vi "TypeDescriptor_SetName.vi"(10 "name":string, 11 "type descriptor":i16[](array[numeric]) format="%04x") -> (1 "named?":bool, 2 "name out":string, 3 "type descriptor dup":i16[](array[numeric]) format="%04x")   [LabVIEW 2013, in "OpenDescriptor.lvlib"]
uses:
  OpenDescriptor.lvlib
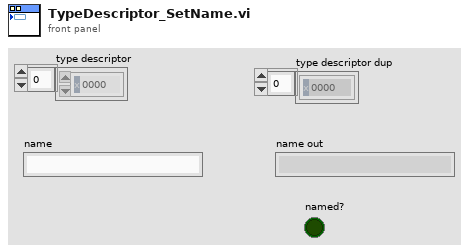
[diagram p1: front panel]
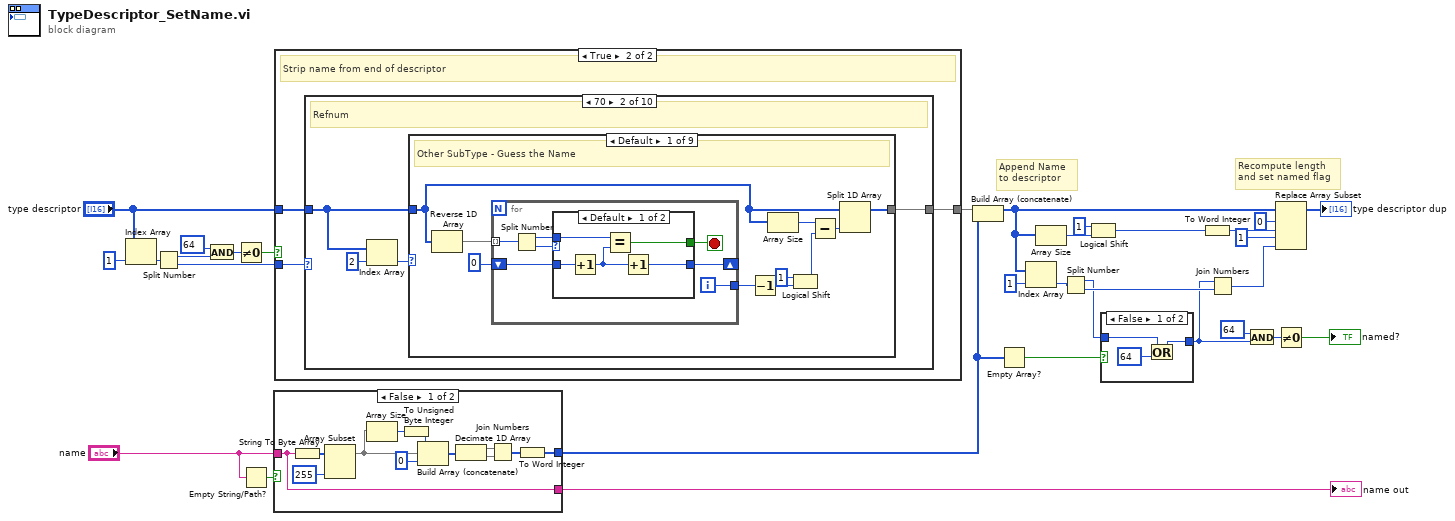
[diagram p0: block diagram]
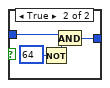
[diagram p2: hidden frame]
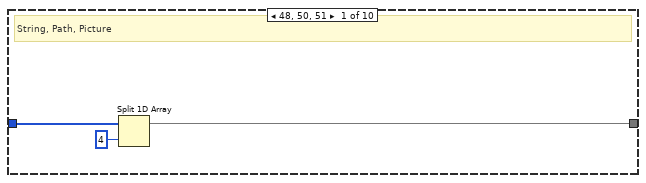
[diagram p5: hidden frame]
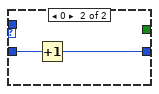
[diagram p6: hidden frame]
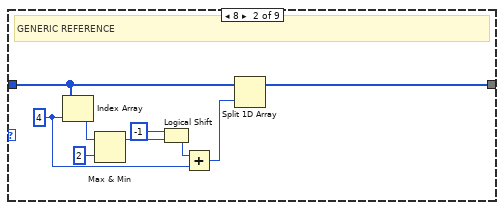
[diagram p7: hidden frame]
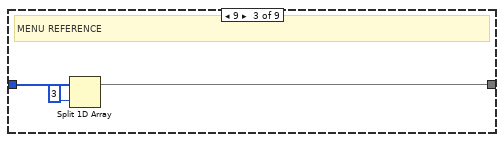
[diagram p8: hidden frame]
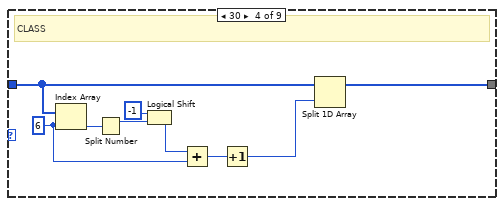
[diagram p9: hidden frame]
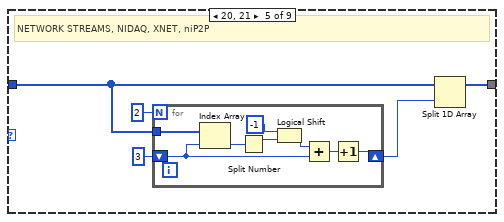
[diagram p10: hidden frame]
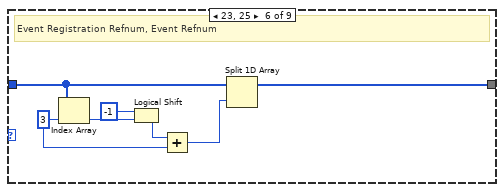
[diagram p11: hidden frame]
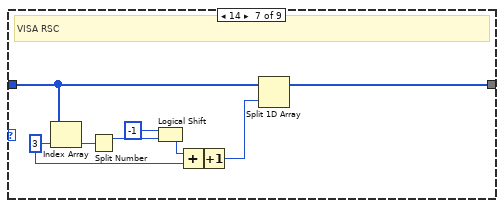
[diagram p12: hidden frame]
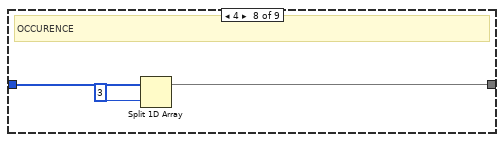
[diagram p13: hidden frame]
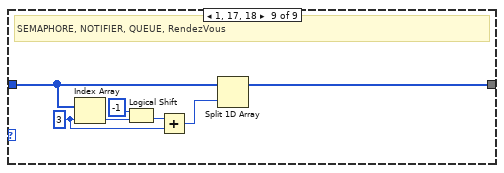
[diagram p14: hidden frame]
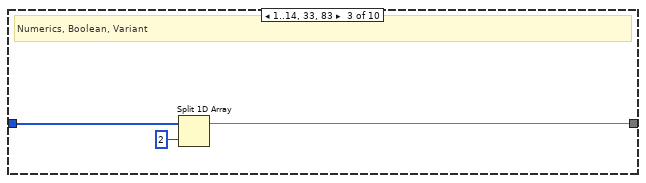
[diagram p15: hidden frame]
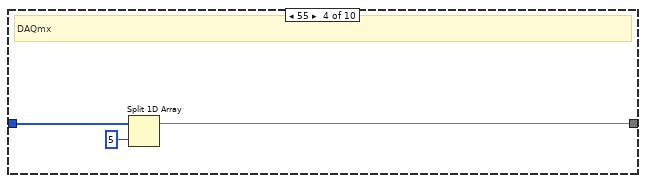
[diagram p16: hidden frame]
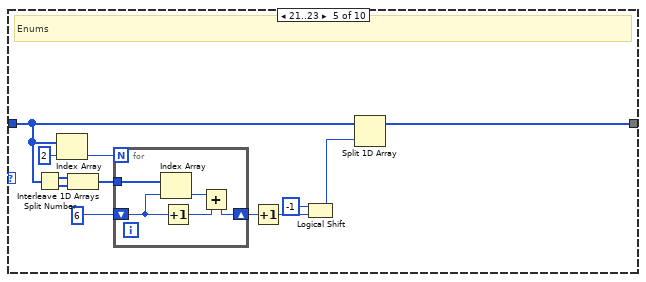
[diagram p17: hidden frame]
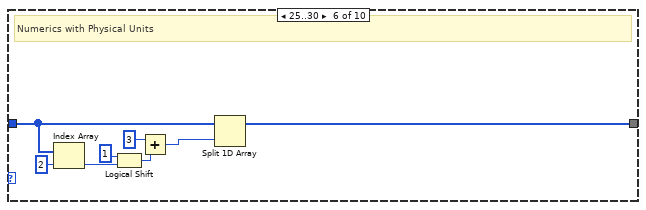
[diagram p18: hidden frame]
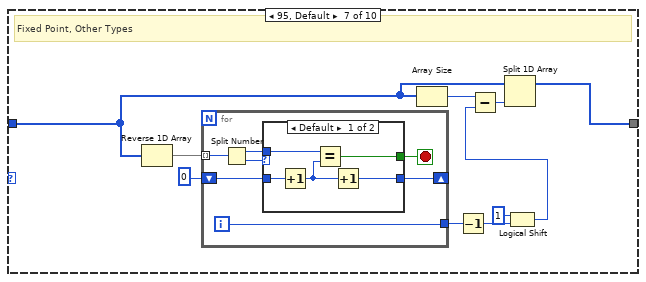
[diagram p19: hidden frame]
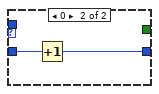
[diagram p20: hidden frame]
diagram:
  # "Recompute length\nand set named flag"
  # "Append Name\nto descriptor"
  n1 = Index Array(array="type descriptor", index=1) -> (element=w31:i16)
  n2 = Split Number(x=w31) -> (hi(x)=w26:u8, lo(x)=w28:u8)
  n3 = And(x=u8 64, y=w26) -> (x .and. y?=w24:u8)
  n4 = Not Equal To 0?(x=w24) -> (x != 0?=w29:bool)
  n5 = Empty String/Path?(string/path="name") -> (empty?=w22:bool)
  n6 = case shown="False" w22 {
    tunnel: [w33 _] -> w8
    tunnel: "name" -> [w32 _]
    tunnel: [w32 _] -> w1
    frame False {
      n7 = String To Byte Array(string=w32) -> (unsigned byte array=w38:u8[])
      n8 = Array Subset(array=w38, length=255) -> (w37:u8[])  [unwired: 1 in]
      n9 = Array Size(array=w37) -> (size(s)=w36:i32)
      n10 = To Unsigned Byte Integer(number=w36) -> (unsigned 8bit integer=w35:u8)
      n11 = Build Array (concatenate)(w35, w37, u8 0) -> (w42:u8[])
      n12 = Decimate 1D Array(w42) -> (w41:u8[], w40:u8[])
      n13 = Join Numbers(hi=w41, lo=w40) -> ((hi.lo)=w34:u16[])
      n14 = To Word Integer(number=w34) -> (16bit integer=w33:i16[])
    }
    frame True {
    }
  }
  "name out" <- w1
  n15 = case shown="True" w29 {
    tunnel: w28 -> [_ w46]
    tunnel: [w44 w45] -> w9
    tunnel: "type descriptor" -> [w44 w47]
    frame False {
    }
    frame True {
      # "Strip name from end of descriptor"
      n16 = case shown="70" w46 {
        tunnel: w47 -> [w50 w52 w140 w143 w147 w164 w174 w195 w207 w215]
        tunnel: [w48 w51 w139 w142 w145 w162 w175 w194 w208 w214] -> w45
        frame 48, 50, 51 {
          # "String, Path, Picture"
          n17 = Split 1D Array(array=w50, index=4) -> (first subarray=w48:i16[])  [unwired: 1 out]
        }
        frame 112 {
          # "Refnum"
          n18 = Index Array(array=w52, index=2) -> (element=w53:i16)
          n19 = case shown="Default" w53 {
            tunnel: w52 -> [w60 w81 w90 w92 w102 w115 w121 w131 w133]
            tunnel: [w59 w79 w88 w91 w101 w113 w122 w129 w132] -> w51
            frame Default {
              # "Other SubType - Guess the Name"
              n20 = Reverse 1D Array(array=w60) -> (reversed array=w63:i16[])
              n21 = for {
                tunnel: w63 -> [w66] mode=indexing
                shift-right: [w68] -> _
                shift-left: u8 0 ("hi(x)") -> [w69]
                tunnel: [w65] -> w55
                i -> [w65]
                stop <- w67 stop-if-true
                n22 = Split Number(x=w66) -> (hi(x)=w70:u8, lo(x)=w71:u8)
                n23 = case shown="Default" w71 {
                  tunnel: [w72 _] -> w67
                  tunnel: w70 -> [w76 _]
                  tunnel: w69 -> [w75 w78]
                  tunnel: [w73 w77] -> w68
                  frame Default {
                    n24 = Increment(x=w75) -> (x+1=w74:u8)
                    n25 = Equal?(x=w76, y=w74) -> (x = y?=w72:bool)
                    n26 = Increment(x=w74) -> (x+1=w73:u8)
                  }
                  frame 0 {
                    n27 = Increment(x=w78) -> (x+1=w77:u8)
                  }
                }
              }
              n28 = Decrement(x=w55) -> (x-1=w57:i32)
              n29 = Array Size(array=w60) -> (size(s)=w62:i32)
              n30 = Logical Shift(y=i16 1, x=w57) -> (x << y=w56:i32)
              n31 = Subtract(x=w62, y=w56) -> (x-y=w61:i32)
              n32 = Split 1D Array(array=w60, index=w61) -> (first subarray=w59:i16[])  [unwired: 1 out]
            }
            frame 8 {
              w85 = 4 ("index")
              # "GENERIC REFERENCE"
              n33 = Index Array(array=w81, index=w85) -> (element=w83:i16)
              n34 = Max & Min(x=w83, y=i16 2) -> (max(x,y)=w84:i16)  [unwired: 1 out]
              n35 = Logical Shift(y=i16 -1, x=w84) -> (x << y=w86:i16)
              n36 = Add(x=w86, y=w85) -> (x+y=w80:i32)
              n37 = Split 1D Array(array=w81, index=w80) -> (first subarray=w79:i16[])  [unwired: 1 out]
            }
            frame 9 {
              # "MENU REFERENCE"
              n38 = Split 1D Array(array=w90, index=3) -> (first subarray=w88:i16[])  [unwired: 1 out]
            }
            frame 30 {
              w95 = 6 ("index")
              # "CLASS"
              n39 = Index Array(array=w92, index=w95) -> (element=w99:i16)
              n40 = Split Number(x=w99) -> (hi(x)=w98:u8)  [unwired: 1 out]
              n41 = Logical Shift(y=i16 -1, x=w98) -> (x << y=w96:u8)
              n42 = Add(x=w96, y=w95) -> (x+y=w94:i32)
              n43 = Increment(x=w94) -> (x+1=w93:i32)
              n44 = Split 1D Array(array=w92, index=w93) -> (first subarray=w91:i16[])  [unwired: 1 out]
            }
            frame 20, 21 {
              # "NETWORK STREAMS, NIDAQ, XNET, niP2P"
              n45 = for {
                N: 2 -> [_]
                shift-right: [w111] -> w100
                shift-left: 3 ("index") -> [w109]
                tunnel: w102 -> [w110]
                n46 = Index Array(array=w110, index=w109) -> (element=w106:i16)
                n47 = Split Number(x=w106) -> (hi(x)=w108:u8)  [unwired: 1 out]
                n48 = Logical Shift(y=i16 -1, x=w108) -> (x << y=w105:u8)
                n49 = Add(x=w105, y=w109) -> (x+y=w112:i32)
                n50 = Increment(x=w112) -> (x+1=w111:i32)
              }
              n51 = Split 1D Array(array=w102, index=w100) -> (first subarray=w101:i16[])  [unwired: 1 out]
            }
            frame 23, 25 {
              w117 = 3 ("index")
              # "Event Registration Refnum, Event Refnum"
              n52 = Index Array(array=w115, index=w117) -> (element=w116:i16)
              n53 = Logical Shift(y=i16 -1, x=w116) -> (x << y=w118:i16)
              n54 = Add(x=w118, y=w117) -> (x+y=w114:i32)
              n55 = Split 1D Array(array=w115, index=w114) -> (first subarray=w113:i16[])  [unwired: 1 out]
            }
            frame 14 {
              w126 = 3 ("index")
              # "VISA RSC"
              n56 = Index Array(array=w121, index=w126) -> (element=w124:i16)
              n57 = Split Number(x=w124) -> (hi(x)=w123:u8)  [unwired: 1 out]
              n58 = Logical Shift(y=i16 -1, x=w123) -> (x << y=w127:u8)
              n59 = Add(x=w127, y=w126) -> (x+y=w125:i32)
              n60 = Increment(x=w125) -> (x+1=w120:i32)
              n61 = Split 1D Array(array=w121, index=w120) -> (first subarray=w122:i16[])  [unwired: 1 out]
            }
            frame 4 {
              # "OCCURENCE"
              n62 = Split 1D Array(array=w131, index=3 ("offset (0)")) -> (first subarray=w129:i16[])  [unwired: 1 out]
            }
            frame 1, 17, 18 {
              w136 = 3 ("index")
              # "SEMAPHORE, NOTIFIER, QUEUE, RendezVous"
              n63 = Index Array(array=w133, index=w136) -> (element=w138:i16)
              n64 = Logical Shift(y=i16 -1, x=w138) -> (x << y=w135:i16)
              n65 = Add(x=w135, y=w136) -> (x+y=w134:i32)
              n66 = Split 1D Array(array=w133, index=w134) -> (first subarray=w132:i16[])  [unwired: 1 out]
            }
          }
        }
        frame 1..14, 33, 83 {
          # "Numerics, Boolean, Variant"
          n67 = Split 1D Array(array=w140, index=2) -> (first subarray=w139:i16[])  [unwired: 1 out]
        }
        frame 55 {
          # "DAQmx"
          n68 = Split 1D Array(array=w143, index=5) -> (first subarray=w142:i16[])  [unwired: 1 out]
        }
        frame 21..23 {
          # "Enums"
          n69 = Split Number(x=w147) -> (hi(x)=w151:u8[], lo(x)=w150:u8[])
          n70 = Index Array(array=w147, index=2) -> (element=w155:i16)
          n71 = Interleave 1D Arrays(w151, w150) -> (w149:u8[])
          n72 = for {
            N: w155 -> [_]
            shift-right: [w159] -> w152
            shift-left: 6 ("index") -> [w158]
            tunnel: w149 -> [w161]
            n73 = Index Array(array=w161, index=w158) -> (element=w160:u8)
            n74 = Increment(x=w158) -> (x+1=w157:i32)
            n75 = Add(x=w160, y=w157) -> (x+y=w159:i32)
          }
          n76 = Increment(x=w152) -> (x+1=w148:i32)
          n77 = Logical Shift(y=i16 -1, x=w148) -> (x << y=w146:i32)
          n78 = Split 1D Array(array=w147, index=w146) -> (first subarray=w145:i16[])  [unwired: 1 out]
        }
        frame 25..30 {
          # "Numerics with Physical Units"
          n79 = Index Array(array=w164, index=2) -> (element=w167:i16)
          n80 = Logical Shift(y=i16 1, x=w167) -> (x << y=w166:i16)
          n81 = Add(x=3, y=w166) -> (x+y=w163:i32)
          n82 = Split 1D Array(array=w164, index=w163) -> (first subarray=w162:i16[])  [unwired: 1 out]
        }
        frame 95, Default {
          # "Fixed Point, Other Types"
          n83 = Reverse 1D Array(array=w174) -> (reversed array=w178:i16[])
          n84 = for {
            tunnel: w178 -> [w181] mode=indexing
            shift-right: [w183] -> _
            shift-left: u8 0 ("hi(x)") -> [w184]
            tunnel: [w180] -> w171
            i -> [w180]
            stop <- w182 stop-if-true
            n85 = Split Number(x=w181) -> (hi(x)=w185:u8, lo(x)=w186:u8)
            n86 = case shown="Default" w186 {
              tunnel: [w187 _] -> w182
              tunnel: w185 -> [w191 _]
              tunnel: w184 -> [w190 w193]
              tunnel: [w188 w192] -> w183
              frame Default {
                n87 = Increment(x=w190) -> (x+1=w189:u8)
                n88 = Equal?(x=w191, y=w189) -> (x = y?=w187:bool)
                n89 = Increment(x=w189) -> (x+1=w188:u8)
              }
              frame 0 {
                n90 = Increment(x=w193) -> (x+1=w192:u8)
              }
            }
          }
          n91 = Array Size(array=w174) -> (size(s)=w177:i32)
          n92 = Decrement(x=w171) -> (x-1=w170:i32)
          n93 = Logical Shift(y=i16 1, x=w170) -> (x << y=w172:i32)
          n94 = Subtract(x=w177, y=w172) -> (x-y=w176:i32)
          n95 = Split 1D Array(array=w174, index=w176) -> (first subarray=w175:i16[])  [unwired: 1 out]
        }
        frame 80 {
          # "Cluster"
          n96 = Index Array(array=w195, index=2) -> (element=w198:i16)
          n97 = for {
            N: w198 -> [_]
            tunnel: w195 -> [w205]
            shift-right: [w200] -> w196
            shift-left: 3 ("index") -> [w201]
            n98 = Index Array(array=w205, index=w201) -> (element=w203:i16)
            n99 = Logical Shift(y=i16 -1, x=w203) -> (x << y=w202:i16)
            n100 = Add(x=w202, y=w201) -> (x+y=w200:i32)
          }
          n101 = Split 1D Array(array=w195, index=w196) -> (first subarray=w194:i16[])  [unwired: 1 out]
        }
        frame 84 {
          # "Waveforms, Timestamp"
          n102 = Index Array(array=w207, index=3) -> (element=w211:i16)
          n103 = Logical Shift(y=i16 -1, x=w211) -> (x << y=w210:i16)
          n104 = Add(x=3 ("y"), y=w210) -> (x+y=w206:i32)
          n105 = Split 1D Array(array=w207, index=w206) -> (first subarray=w208:i16[])  [unwired: 1 out]
        }
        frame 64 {
          # "Arrays"
          n106 = Index Array(array=w215, index=2) -> (element=w220:i16)
          n107 = Logical Shift(y=i16 1, x=w220) -> (x << y=w219:i16)
          n108 = Add(x=w219, y=3) -> (x+y=w218:i32)
          n109 = Index Array(array=w215, index=w218) -> (element=w221:i16)
          n110 = Logical Shift(y=i16 -1, x=w221) -> (x << y=w217:i16)
          n111 = Add(x=w217, y=w218) -> (x+y=w216:i32)
          n112 = Split 1D Array(array=w215, index=w216) -> (first subarray=w214:i16[])  [unwired: 1 out]
        }
      }
    }
  }
  n113 = Build Array (concatenate)(w9, w8) -> (w17:i16[])
  n114 = Empty Array?(array=w8) -> (empty?=w7:bool)
  n115 = Index Array(array=w17, index=1) -> (element=w18:i16)
  n116 = Array Size(array=w17) -> (size(s)=w11:i32)
  n117 = Split Number(x=w18) -> (hi(x)=w6:u8, lo(x)=w19:u8)
  n118 = Logical Shift(y=i16 1, x=w11) -> (x << y=w14:i32)
  n119 = case shown="False" w7 {
    tunnel: w6 -> [w227 w230]
    tunnel: [w228 w229] -> w3
    frame False {
      n120 = Or(x=w227, y=u8 64 ("x")) -> (x .or. y?=w228:u8)
    }
    frame True {
      n121 = Not(x=u8 64) -> (.not. x?=w232:u8)
      n122 = And(x=w230, y=w232) -> (x .and. y?=w229:u8)
    }
  }
  n123 = To Word Integer(number=w14) -> (16bit integer=w15:i16)
  n124 = Join Numbers(hi=w3, lo=w19) -> ((hi.lo)=w21:u16)
  n125 = And(x=u8 64, y=w3) -> (x .and. y?=w5:u8)
  n126 = Replace Array Subset(array=w17, new element #1=w15, index #1=0 ("index"), new element #2=w21, index #2=1 ("index")) -> (→"type descriptor dup":i16[])
  n127 = Not Equal To 0?(x=w5) -> (x != 0?=→"named?":bool)
